vi "CompressorSoundPlay.vi"() -> ()   [LabVIEW 2014]
panel:
  out "Numeric":i32
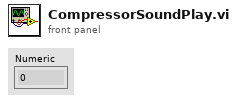
[diagram p1: front panel]
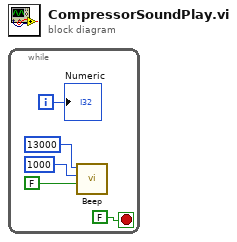
[diagram p0: block diagram]
diagram:
  n1 = while {
    i -> [w3]
    stop <- FALSE stop-if-true
    n2 = call <vilib>:"Beep.vi"("use system alert? (T)"=FALSE, "duration (msec)"=u32 1000, "frequency (Hz)"=u32 13000) -> ()  [unwired: 9 in]
    "Numeric" <- w3
  }
